vi "MASZYNA FINAL pmp.vi"(0 "F max":dbl, 4 "Rozpocznij":bool, 5 "F min":dbl, 6 "Zatrzymaj":bool, 7 "Ilosc probek":u32, 8 "Wyjście":bool, 9 "Amplituda":dbl, 10 "Zapisz":bool, 11 "Włącz":bool, 13 "X LIN/LOG":bool, 14 "Y LIN/LOG":bool, 15 "Wybór obiektu":u32(slide)=1 scale=1.0..4.0) -> (1 "V out":dbl[](array[numeric]), 2 "V in":dbl[](array[numeric]), 3 "Częstotliwosc":dbl[](array[numeric]), 12 "V out / V in":dbl[](array[numeric]))   [LabVIEW 2021]
doc: "maszyna stanów obsługująca projekt\nprosze o 3.0\n:3"
uses:
  controlmaszyna.ctl
  <vilib>/Utility/file.llb/Write Delimited Spreadsheet (string).vi
panel:
  out "XY Graph":cluster{"Częstotliwosc":dbl[], dbl[]}(graph)
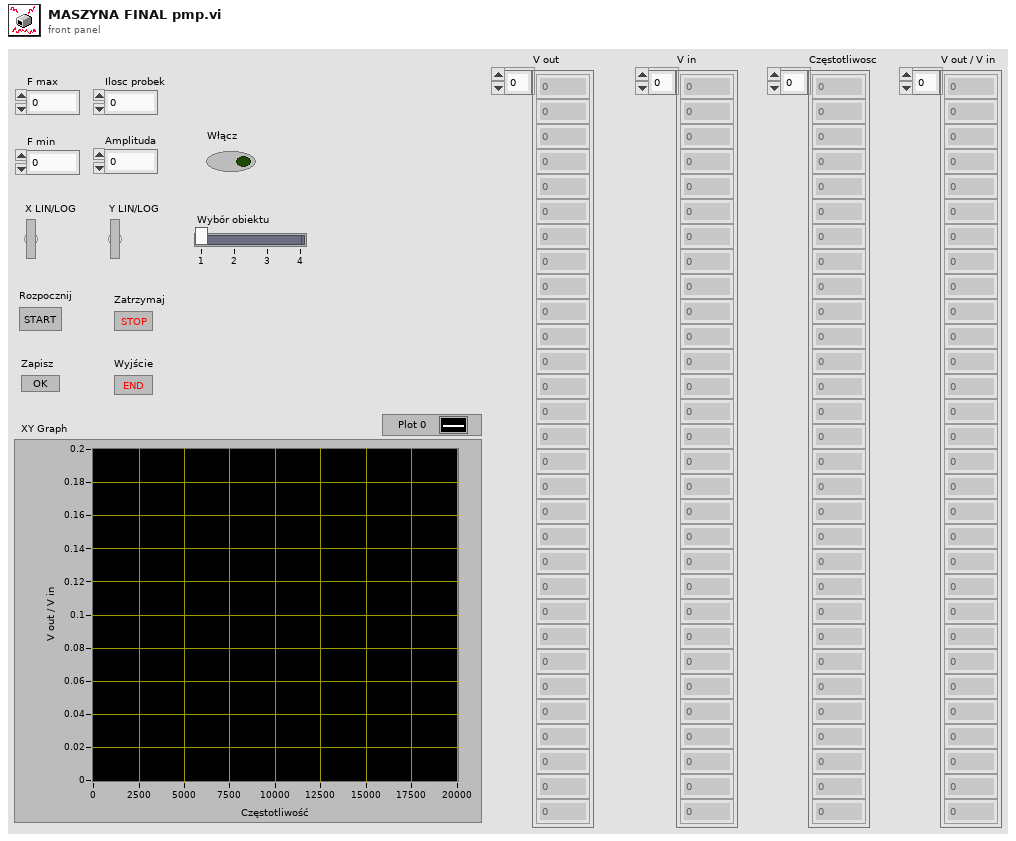
[diagram p1: front panel]
types:
  T1 = typedef "controlmaszyna.ctl" = enum16{"init", "praca", "pomiar", "wykres", "zapis", "stop", "koniec"}
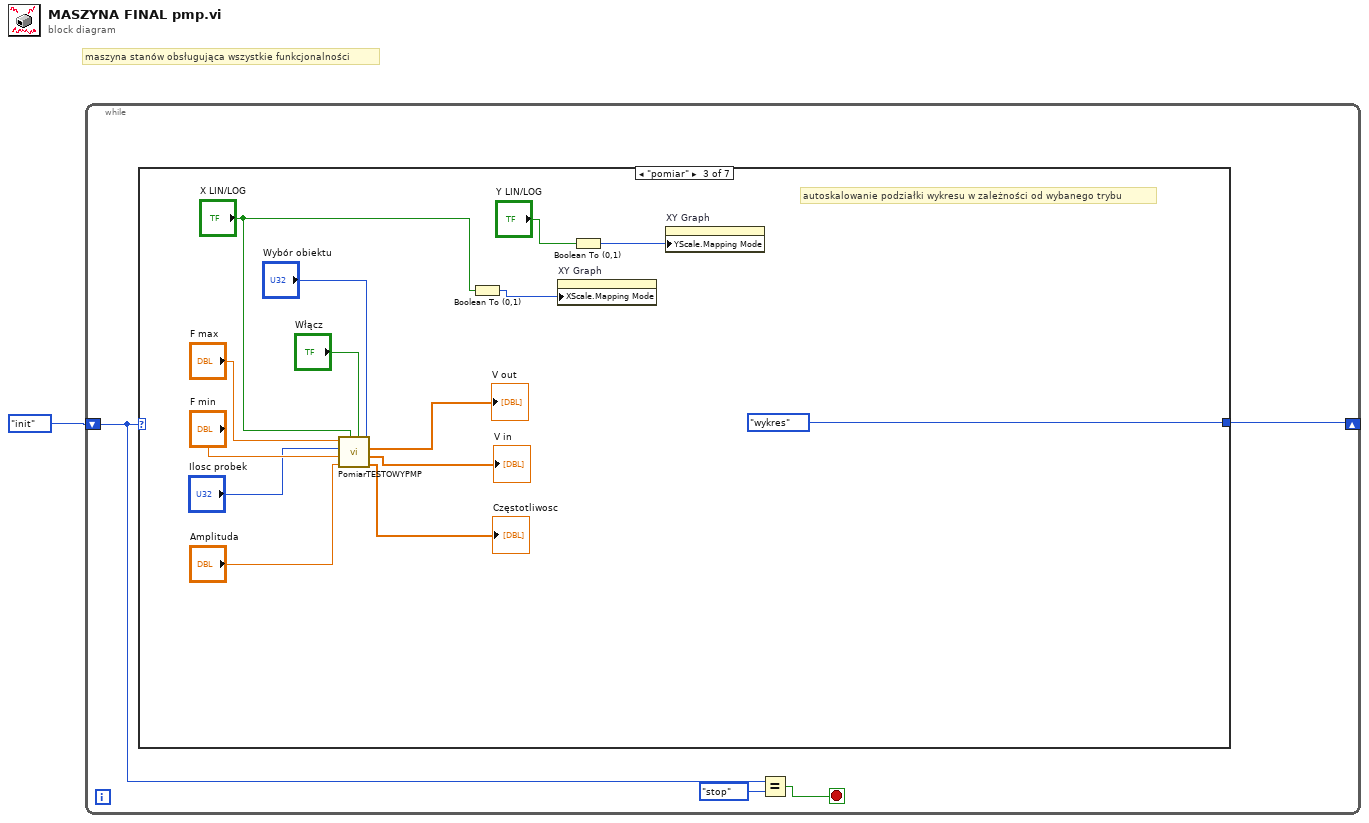
[diagram p0: block diagram]
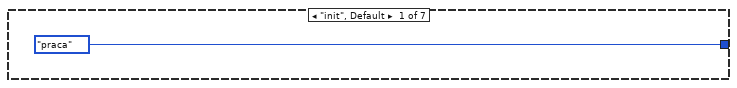
[diagram p2: hidden frame]
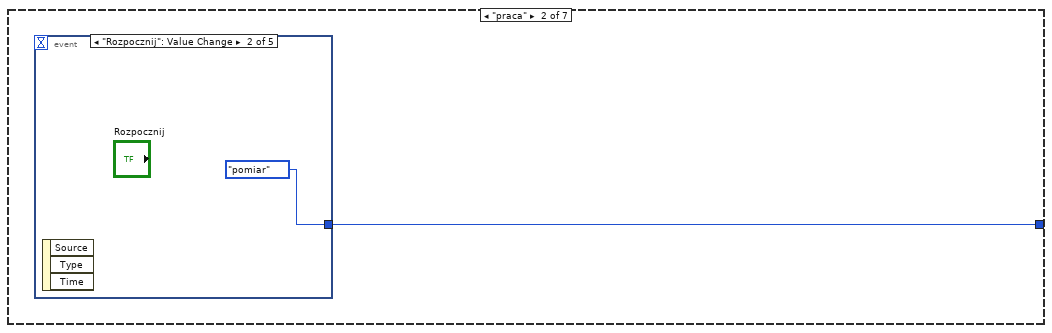
[diagram p3: hidden frame]
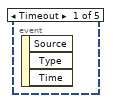
[diagram p4: hidden frame]
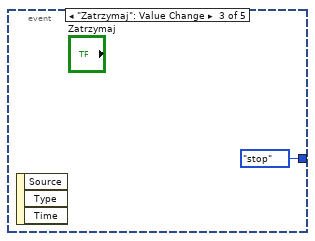
[diagram p5: hidden frame]
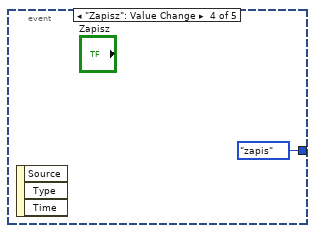
[diagram p6: hidden frame]
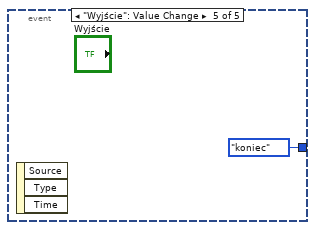
[diagram p7: hidden frame]
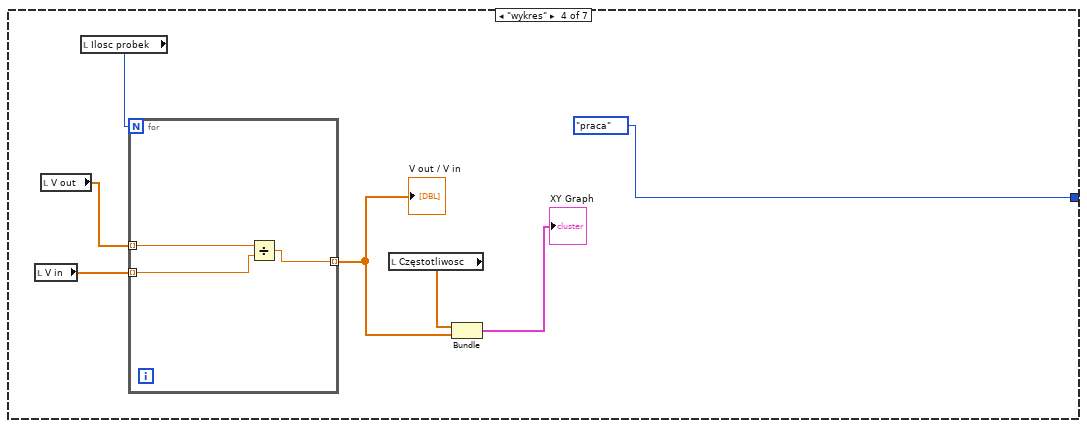
[diagram p8: hidden frame]
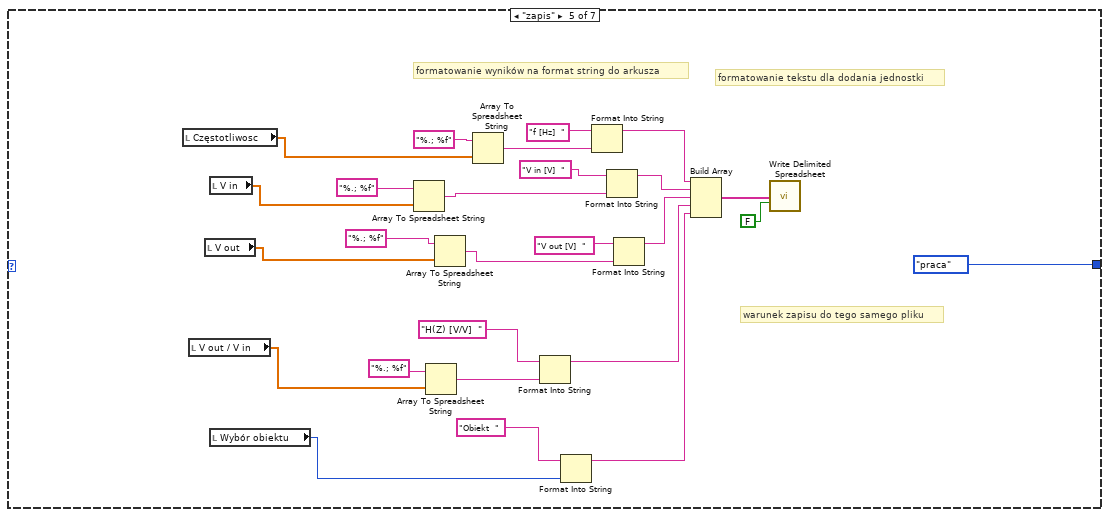
[diagram p9: hidden frame]
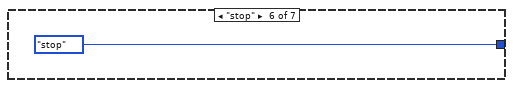
[diagram p10: hidden frame]
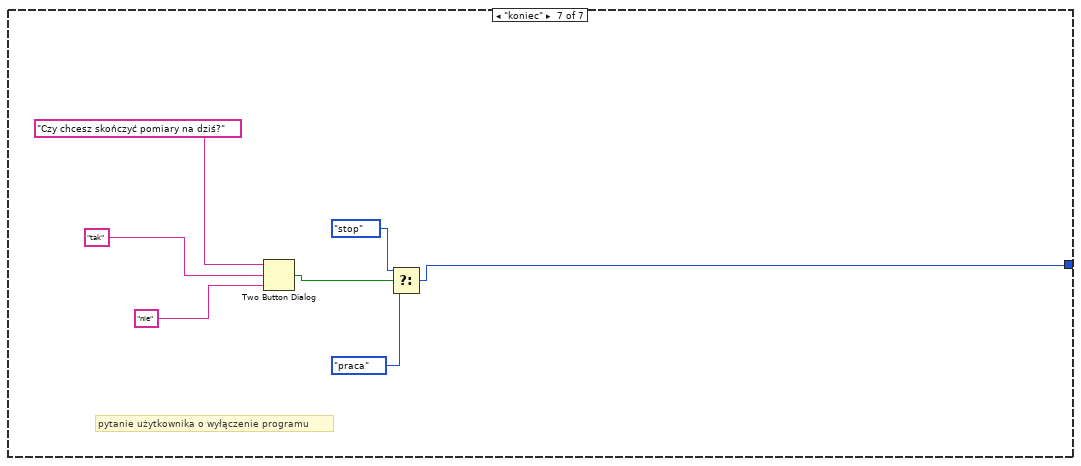
[diagram p11: hidden frame]
diagram:
  # "maszyna stanów obsługująca wszystkie funkcjonalności"
  n1 = while {
    shift-right: [w5] -> _
    shift-left: controlmaszyna."init" -> [w4]
    stop <- w2 stop-if-true
    n2 = case shown="\"pomiar\"" w4 {
      tunnel: [controlmaszyna."praca" w7 controlmaszyna."wykres" controlmaszyna."praca" controlmaszyna."praca" controlmaszyna."stop" w63] -> w5
      frame "init", Default {
      }
      frame "praca" {
        n3 = event shown="[1] \"Rozpocznij\": Value Change" {
          selector: _ -> [_ _ _ _ _]
          dyn-events: _ -> [_ _ _ _ _]
          timeout: _ -> [_ _ _ _ _]
          tunnel: [_ controlmaszyna."pomiar" controlmaszyna."stop" controlmaszyna."zapis" controlmaszyna."koniec"] -> w7
          event Timeout {
            n4 = event-data() -> ()  [unwired: 1 in, 3 out]
          }
          event "Rozpocznij": Value Change {
            n5 = event-data() -> ()  [unwired: 1 in, 3 out]
          }
          event "Zatrzymaj": Value Change {
            n6 = event-data() -> ()  [unwired: 1 in, 3 out]
          }
          event "Zapisz": Value Change {
            n7 = event-data() -> ()  [unwired: 1 in, 3 out]
          }
          event "Wyjście": Value Change {
            n8 = event-data() -> ()  [unwired: 1 in, 3 out]
          }
        }
      }
      frame "pomiar" {
        # "autoskalowanie podziałki wykresu w zależności od wybanego trybu"
        n9 = call "PomiarTESTOWYPMP.vi"("Wybór obiektu"="Wybór obiektu", "WLACZ"="Włącz", "Liniowy/Logarytmiczny"="X LIN/LOG", "Amplituda"="Amplituda", "F min"="F min", "ilosc probek"="Ilosc probek", "F max"="F max") -> ("Czestotliwosc"=→"Częstotliwosc":dbl[], "V in"=→"V in":dbl[], "V out"=→"V out":dbl[])
        n10 = Boolean To (0,1)(Boolean="X LIN/LOG") -> (0, 1=w23:i16)
        n11 = property on="XY Graph" class="XYGraph (strict)"("XScale.Mapping Mode"=w23) -> ()  [unwired: 2 in, 2 out]
        n12 = Boolean To (0,1)(Boolean="Y LIN/LOG") -> (0, 1=w24:i16)
        n13 = property on="XY Graph" class="XYGraph (strict)"("YScale.Mapping Mode"=w24) -> ()  [unwired: 2 in, 2 out]
      }
      frame "wykres" {
        n14 = local read "V in"() -> (w30:dbl[])
        n15 = local read "V out"() -> (w31:dbl[])
        n16 = local read "Ilosc probek"() -> (w32:u32)
        n17 = for {
          N: w32 -> [_]
          tunnel: w31 -> [w35] mode=indexing
          tunnel: w30 -> [w34] mode=indexing
          tunnel: [w33] -> w29 mode=indexing
          n18 = Divide(x=w35, y=w34) -> (x/y=w33:dbl)
        }
        "V out / V in" <- w29
        n19 = local read "Częstotliwosc"() -> (w28:dbl[])
        n20 = Bundle("Częstotliwosc"=w28, w29) -> (→"XY Graph":cluster{"Częstotliwosc":dbl[], dbl[]})  [unwired: 1 in]
      }
      frame "zapis" {
        # "warunek zapisu do tego samego pliku"
        # "formatowanie tekstu dla dodania jednostki"
        # "formatowanie wyników na format string do arkusza"
        n21 = local read "Częstotliwosc"() -> (w40:dbl[])
        n22 = local read "V out / V in"() -> (w37:dbl[])
        n23 = local read "V out"() -> (w38:dbl[])
        n24 = local read "V in"() -> (w39:dbl[])
        n25 = local read "Wybór obiektu"() -> (w36:u32)
        n26 = Array To Spreadsheet String(array=w39, 3:"%.; %f" ("format string")) -> (spreadsheet string=w52:string)  [unwired: 1 in]
        n27 = Array To Spreadsheet String(array=w37, 3:"%.; %f" ("format string")) -> (spreadsheet string=w54:string)  [unwired: 1 in]
        n28 = Array To Spreadsheet String(array=w38, 3:"%.; %f" ("format string")) -> (spreadsheet string=w50:string)  [unwired: 1 in]
        n29 = Array To Spreadsheet String(array=w40, 3:"%.; %f" ("format string")) -> (spreadsheet string=w56:string)  [unwired: 1 in]
        n30 = Format Into String(initial string="H(Z) [V/V]  ", w54) -> (resulting string=w43:string)  [unwired: 2 in, 1 out]
        n31 = Format Into String(initial string="Obiekt  ", w36) -> (resulting string=w41:string)  [unwired: 2 in, 1 out]
        n32 = Format Into String(initial string="f [Hz]  " ("element"), w56) -> (resulting string=w46:string)  [unwired: 2 in, 1 out]
        n33 = Format Into String(initial string="V in [V]  " ("element"), w52) -> (resulting string=w45:string)  [unwired: 2 in, 1 out]
        n34 = Format Into String(initial string="V out [V]  " ("element"), w50) -> (resulting string=w44:string)  [unwired: 2 in, 1 out]
        n35 = Build Array(w46, w45, w44, w43, w41) -> (w59:string[])
        n36 = call-poly <vilib>:"Write Delimited Spreadsheet.vi"("1D data"=w59, "append to file? (new file:F)"=FALSE) -> ()  [unwired: 12 in, 2 out]
      }
      frame "stop" {
      }
      frame "koniec" {
        # "pytanie użytkownika o wyłączenie programu"
        n37 = Two Button Dialog(message="Czy chcesz skończyć pomiary na dziś?", 1:"nie" ("F button name (\"Cancel\")"), 2:"tak" ("T button name (\"OK\")")) -> (T button?=w66:bool)
        n38 = Select(t=controlmaszyna."stop", s=w66, f=controlmaszyna."praca") -> (s? t:f=w63:T1)
      }
    }
    n39 = Equal?(x=w4, y=controlmaszyna."stop") -> (x = y?=w2:bool)
  }
